vi "CR slave_Create.vi"(8 "error in (no error)":errorcluster, 10 "ID":string, 11 "reference in":refnum<class "CR slave.lvclass">) -> (0 "error out":errorcluster, 3 "reference out":refnum<class "CR slave.lvclass">)   [LabVIEW 2019, in "CommandResponse communication.lvlib" / "CR slave.lvclass"]
doc: "Constructor."
uses:
  CR slave.lvclass
  C:/Program Files/National Instruments/LabVIEW 2019/vi.lib/addons/_AddQ/G#Object/G#Object.lvclass
  <vilib>/addons/_AddQ/G#Object/G#Object.lvclass
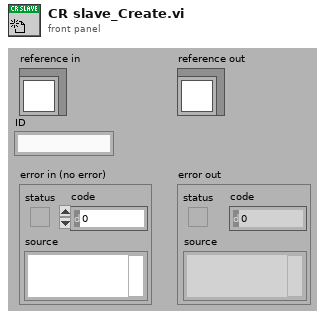
[diagram p1: front panel]
types:
  T1 = typedef "CommandResponse communication.lvlib/CR slave.lvclass/ObjectAttributesRef.ctl" = refnum<data-value>
  T2 = typedef "CommandResponse communication.lvlib/CR slave.lvclass/ObjectAttributes.ctl" = cluster{"connected":bool, "stop":bool, "ID":string}
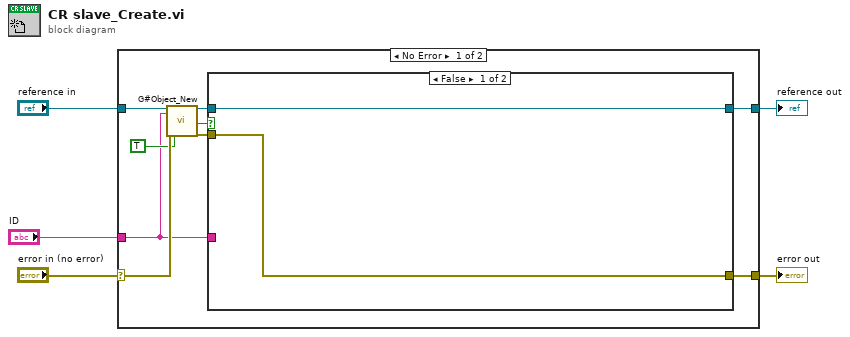
[diagram p0: block diagram]
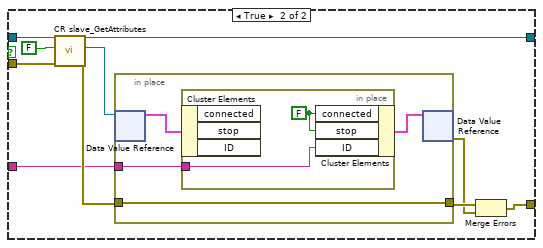
[diagram p2: hidden frame]
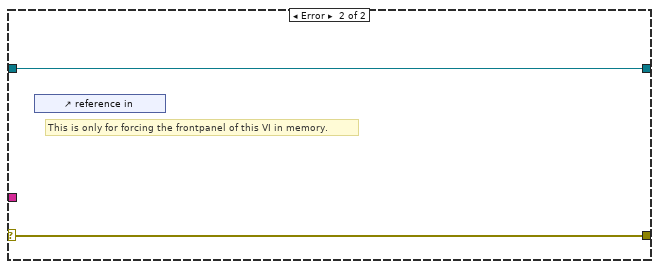
[diagram p3: hidden frame]
diagram:
  n1 = case shown="No Error" "error in (no error)" {
    selector: "error in (no error)" -> [w13 w34]
    tunnel: [w12 w34] -> w4
    tunnel: [w9 w33] -> w2
    tunnel: "reference in" -> [w14 w33]
    tunnel: "ID" -> [w7 _]
    frame No Error {
      n2 = call <vilib>:"G#Object_New.vi"("reference in"=w14, "object name"=w7, "error in (no error)"=w13, "user counter (T)?"=TRUE ("User Counter")) -> ("reference out"=w10:refnum<class "CR slave.lvclass">, "created new?"=w6:bool, "error out"=w8:errorcluster)  [unwired: 13 in]
      n3 = case shown="False" w6 {
        tunnel: [w15 w26] -> w12
        tunnel: w10 -> [w16 w23]
        tunnel: [w16 w22] -> w9
        tunnel: w8 -> [w15 w21]
        tunnel: w7 -> [_ w17]
        frame False {
        }
        frame True {
          n4 = call "CR slave_GetAttributes.vi"("error in (no error)"=w21, "return data? (T)"=FALSE ("return data"), "reference in"=w23) -> ("error out"=w20:errorcluster, "attributes ref"=w19:T1, "reference out"=w22:refnum<class "CR slave.lvclass">)  [unwired: 5 in, 1 out]
          n5 = in-place {
            in-place-border: w20 -> [w28]
            in-place-border: [w28] -> w25
            in-place-border: w17 -> [w27]
            n6 = in-place-dvr #1(w19) -> (w29:T2)  [unwired: 1 out]
            n7 = in-place {
              in-place-border: w27 -> [w31]
              w32 = FALSE ("connected")
              n8 = in-place-cluster #2(w29) -> ()  [unwired: 3 out]
              n9 = in-place-cluster #2("connected"=w32, "stop"=w32, "ID"=w31) -> (w30:T2)
            }
            n10 = in-place-dvr #1(w30) -> (w24:errorcluster)  [unwired: 1 out]
          }
          n11 = Merge Errors(w25, w24) -> (w26:errorcluster)
        }
      }
    }
    frame Error {
      # "This is only for forcing the frontpanel of this VI in memory."
      n12 = control-ref of="reference in"() -> ()  [unwired: 1 out]
    }
  }
  "error out" <- w4
  "reference out" <- w2
